vi "ABCtoDQ_3PhaseUnitaryMagnitude_src.vi"(0 "A":sgl, 5 "B":sgl, 7 "C":sgl, 9 "Theta":sgl) -> (4 "direct":sgl, 6 "quadrature":sgl, 8 "alpha":sgl, 10 "beta":sgl, 13 "sinx":sgl, 14 "cosx":sgl)   [LabVIEW 2017]
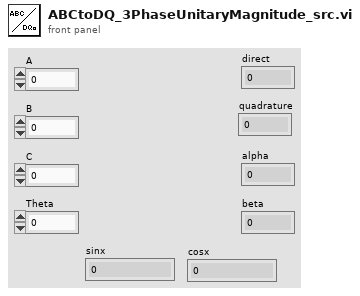
[diagram p1: front panel]
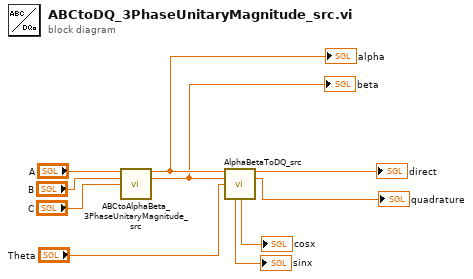
[diagram p0: block diagram]
diagram:
  n1 = call "ABCtoAlphaBeta_3PhaseUnitaryMagnitude_src.vi"("A"="A", "B"="B", "C"="C") -> ("alpha"=w10:sgl, "beta"=w9:sgl)  [unwired: 11 in]
  "alpha" <- w10
  "beta" <- w9
  n2 = call "AlphaBetaToDQ_src.vi"("alpha"=w10, "beta"=w9, "theta"="Theta") -> ("direct"=→"direct":sgl, "quadrature"=→"quadrature":sgl, "sinx"=→"sinx":sgl, "cosx"=→"cosx":sgl)  [unwired: 9 in]
